vi "Send command Set Port.vi"(7 "Marca":string, 8 "error in (no error)":errorcluster, 9 "Valor HEX":string, 10 "Puerto":string, 11 "Simulado in":refnum<class "Simulado.lvclass">) -> (0 "error out":errorcluster, 1 "Command":string, 2 "Expected response":string, 3 "Simulado out":refnum<class "Simulado.lvclass">)   [LabVIEW 2020, in "Simulado.lvclass"]
doc: "Se manda el comando para poner el peurto en un valor en hexadecimal, se escribe en el puerto serial y se lee la respuesta que de el micro."
uses:
  Simulado.lvclass
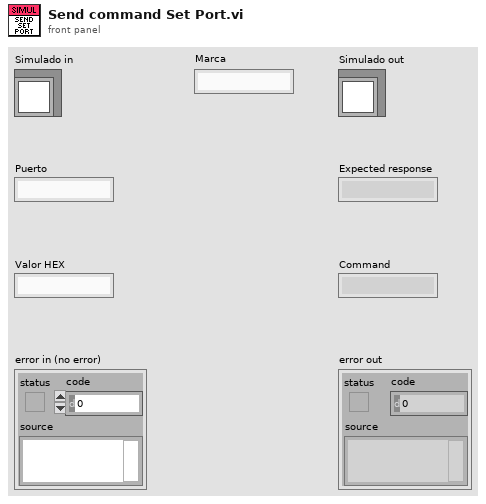
[diagram p1: front panel]
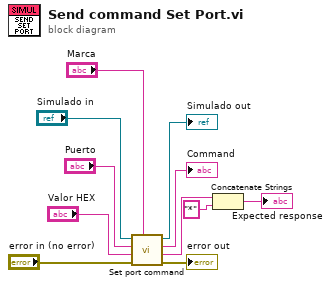
[diagram p0: block diagram]
diagram:
  n1 = call-dynamic "Set port command.vi"("Marca"="Marca", "error in (no error)"="error in (no error)", "Valor HEX"="Valor HEX", "Puerto"="Puerto", "Serial Device in"="Simulado in") -> ("error out"=→"error out":errorcluster, "Expected response"=w1:string, "Command"=→"Command":string, "Serial Device out"=→"Simulado out":refnum<class "Simulado.lvclass">)  [unwired: 3 in]
  n2 = Concatenate Strings(w1, "*" ("string")) -> (→"Expected response":string)
